vi "Read RunningAveragePeriodSettings.vi"(8 "error in (no error)":errorcluster, 11 "RunningAverageCalculation in":refnum<class "RunningAverageCalculation.lvclass">) -> (0 "error out":errorcluster, 2 "RunningAveragePeriodSettings":dbl[](array[numeric]), 3 "RunningAverageCalculation out":refnum<class "RunningAverageCalculation.lvclass">)   [LabVIEW 2015, in "RunningAverageCalculation.lvclass"]
uses:
  RunningAverageCalculation.lvclass
  RunningAverageCalculation.lvclass/RunningAverageCalculation.ctl
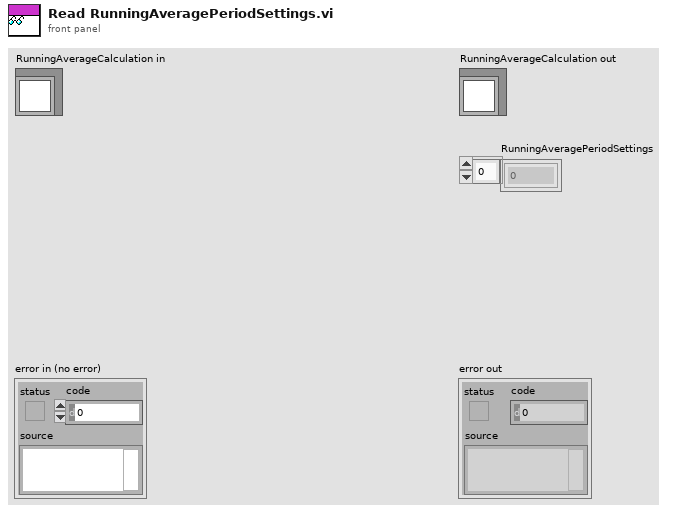
[diagram p1: front panel]
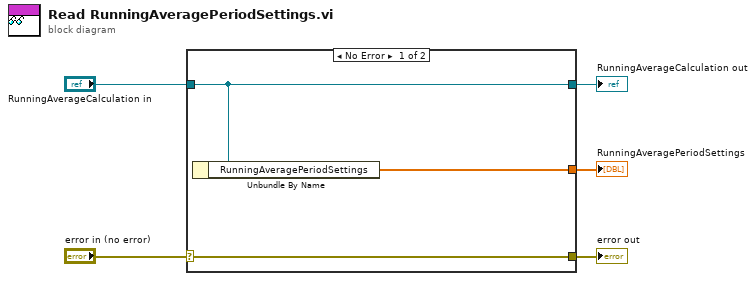
[diagram p0: block diagram]
diagram:
  n1 = case shown="No Error" "error in (no error)" {
    selector: "error in (no error)" -> [w8 w9]
    tunnel: [w8 w9] -> w4
    tunnel: [w7 w10] -> w2
    tunnel: "RunningAverageCalculation in" -> [w7 w10]
    tunnel: [w6 _] -> w1
    frame No Error {
      n2 = Unbundle By Name(w7) -> ("RunningAveragePeriodSettings"=w6:dbl[])
    }
    frame Error {
    }
  }
  "error out" <- w4
  "RunningAverageCalculation out" <- w2
  "RunningAveragePeriodSettings" <- w1
